vi "Load Reference.vi"(8 "error in (no error)":errorcluster, 10 "Reference":refnum<vi>, 11 "Cleaningcycle in":refnum<class "Cleaning cycle.lvclass">) -> (0 "error out":errorcluster, 3 "Cleaningcycle out":refnum<class "Cleaning cycle.lvclass">)   [LabVIEW 2016, in "Cleaning cycle.lvclass"]
doc: "The <b>Load Reference VI</b> is a dynamic dispatch VI that must be overwritten in every QControl Class and must <b>Call Parent Method</b>. This recursively loads the reference of the control to the data space for the Control Class up the inheritance hierarchy (class hierarchy). These references must be loaded in this way to use all of the built-in properties.\n\nThe reference input is the reference type needed for the control but is coerced to Generic. It should be cast back to the correct type before bundling into the class private data. The pre-casted \"Generic\" reference is wired as input to the <b>Call Parent Method</b>.\n<b> </b> <b> </b>\n©2016 Q Software Innovations, LLC (QSI)\nwritten by Quentin Alldredge\nproduced in LabVIEW 2015\n\nsupport@qsoftwareinnovations.com\nwww.qsoftwareinnovations.com\n\nAll rights reserved.\n\nRedistribution and use in source and binary forms, with or without modification, are permitted provided that the following conditions are met:\n\n * Redistributions of source code must retain the above copyright notice, this list of conditions and the following disclaimer.\n * Redistributions in binary form must reproduce the above copyright notice, this list of conditions and the following disclaimer in the documentation and/or other materials provided with the distribution.\n * Neither the name of Q Software Innovations, LLC. nor the names of its contributors may be used to endorse or promote products derived from this software without specific prior written permission.\n\nTHIS SOFTWARE IS PROVIDED BY THE COPYRIGHT HOLDERS AND CONTRIBUTORS \"AS IS\" AND ANY EXPRESS OR IMPLIED WARRANTIES, INCLUDING, BUT NOT LIMITED TO, THE IMPLIED WARRANTIES OF MERCHANTABILITY AND FITNESS FOR A PARTICULAR PURPOSE ARE DISCLAIMED. IN NO EVENT SHALL THE COPYRIGHT OWNER OR CONTRIBUTORS BE LIABLE FOR ANY DIRECT, INDIRECT, INCIDENTAL, SPECIAL, EXEMPLARY, OR CONSEQUENTIAL DAMAGES (INCLUDING, BUT NOT LIMITED TO, PROCUREMENT OF SUBSTITUTE GOODS OR SERVICES; LOSS OF USE, DATA, OR PROFITS; OR BUSINESS INTERRUPTION) HOWEVER CAUSED AND ON ANY THEORY OF LIABILITY, WHETHER IN CONTRACT, STRICT LIABILITY, OR TORT (INCLUDING NEGLIGENCE OR OTHERWISE) ARISING IN ANY WAY OUT OF THE USE OF THIS SOFTWARE, EVEN IF ADVISED OF THE POSSIBILITY OF SUCH DAMAGE."
uses:
  Cleaning cycle.lvclass
  Cleaning cycle.lvclass/Cleaning cycle.ctl
  <vilib>/QSI/QControls/QControl Classes/Cluster/Cluster.lvclass
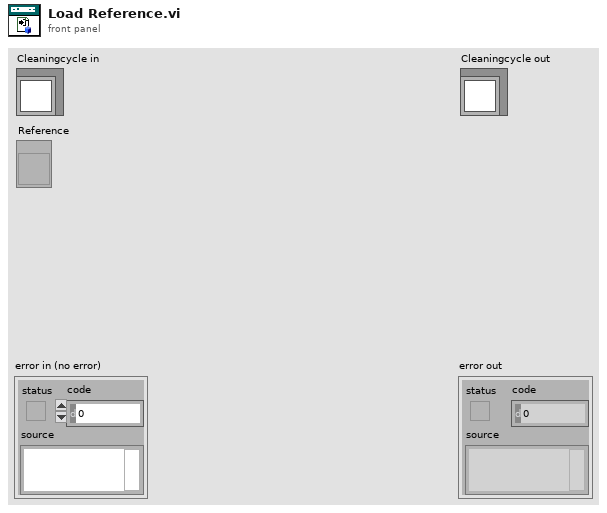
[diagram p1: front panel]
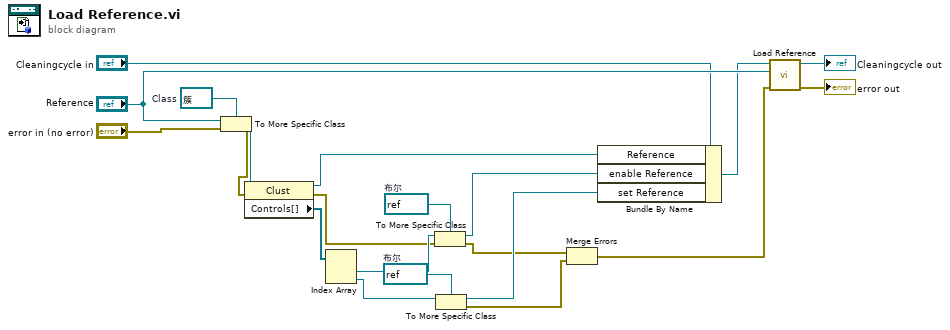
[diagram p0: block diagram]
diagram:
  w7 = refnum<vi> refnum  # 布尔
  w8 = refnum<vi> refnum  # 布尔
  w20 = refnum<vi> refnum  # Class
  n1 = To More Specific Class(target class=w20, reference="Reference", error in="error in (no error)") -> (specific class reference=w14:refnum<vi>, error out=w9:errorcluster)
  n2 = property class="Clust"(reference=w14, error in=w9) -> (reference out=w13:refnum<vi>, error out=w10:errorcluster, "Controls[]"=w12:refnum<vi>[])
  n3 = Index Array(array=w12) -> (element #1=w11:refnum<vi>, element #2=w1:refnum<vi>)  [unwired: 2 in]
  n4 = To More Specific Class(target class=w8, reference=w11, error in=w10) -> (specific class reference=w6:refnum<vi>, error out=w4:errorcluster)
  n5 = To More Specific Class(target class=w7, reference=w1) -> (specific class reference=w5:refnum<vi>, error out=w3:errorcluster)  [unwired: 1 in]
  n6 = Merge Errors(w4, w3) -> (w2:errorcluster)
  n7 = Bundle By Name(cluster="Cleaningcycle in", "Reference"=w13, "enable Reference"=w6, "set Reference"=w5) -> (w19:refnum<class "Cleaning cycle.lvclass">)
  n8 = call-parent "Load Reference.vi"("error in (no error)"=w2, "Reference"="Reference", "Cluster in"=w19) -> ("error out"=→"error out":errorcluster, "Cluster out"=→"Cleaningcycle out":refnum<class "Cleaning cycle.lvclass">)  [unwired: 7 in]
